vi "mb Convert [U8] to U16.vi"(2 "Data [ ]":u8[](array[numeric]), 4 "Byte Offset":u16=1) -> (6 "U16 Data [ ]":u16[](array[numeric]), 7 "U16 Data":u16)   [LabVIEW 2009]
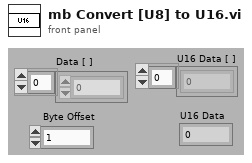
[diagram p1: front panel]
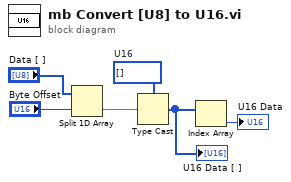
[diagram p0: block diagram]
diagram:
  w2 = u16[] []  # U16
  n1 = Split 1D Array(array="Data [ ]", index="Byte Offset") -> (second subarray=w3:u8[])  [unwired: 1 out]
  n2 = Type Cast(type=w2, x=w3) -> (*(type *) &x=w1:u16[])
  "U16 Data [ ]" <- w1
  n3 = Index Array(array=w1) -> (element=→"U16 Data":u16)  [unwired: 1 in]
